vi "Pack for gRPC.vi"(8 "error in":errorcluster, 9 "configuration / results":enum16{"Configuration", "Results"}(ring), 10 "data value":variant, 11 "measurement plugin in":refnum<class "FPT Intermodulation.lvclass">) -> (0 "error out":errorcluster, 2 "any":T1, 3 "measurement plugin out":refnum<class "FPT Intermodulation.lvclass">)   [LabVIEW 2023, in "FPT Intermodulation.lvclass"]
uses:
  FPT Intermodulation.lvclass
  <vilib>/gRPC/LabVIEW gRPC Library/Shared/Any.ctl
  C:/Program Files/National Instruments/LabVIEW 2023/vi.lib/Plug-In SDKs/Measurements/Measurement Plugin Service/Measurement Plugin Service.lvclass
  Measurement Configuration.ctl
  Measurement Results.ctl
  2eca732d-dbaa-43bf-a7dd-ede2da65bc1b.vi
  a6012965-5700-4384-8228-972e71b6560c.vi
  <vilib>/gRPC/LabVIEW gRPC Library/Server API/Translate Protobuf Error.vi
  <vilib>/AdvancedString/1D String Array to Delimited String.vi
  <vilib>/gRPC/LabVIEW gRPC Library/Server API/Server/Get Server DLL Path.vi
  <vilib>/Plug-In SDKs/Measurements/Measurement Plugin Service/Measurement Plugin Service.lvclass
  <vilib>/gRPC/LabVIEW gRPC Library/grpc-lvsupport-release.lvlib
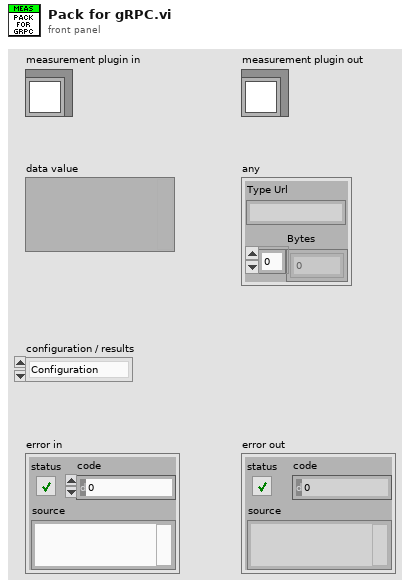
[diagram p1: front panel]
types:
  T1 = typedef "grpc-lvsupport-release.lvlib/Any.ctl" = cluster{"Type Url":string, "Bytes":u8[]}
  T2 = typedef "grpc-lvsupport-release.lvlib/grpcId.ctl" = u64
  T3 = typedef "FPT Intermodulation.lvclass/Measurement Configuration.ctl" = cluster{"Automation Test":bool, "Power sequencing file path":string, "RFSG name":string, "RFSG port":string, "RFSG attenuation mode":enum32{"<None>", "Constant Attenuation", "s2p File"}, "RFSG external attenuation (dB)":dbl, "RFSG s-parameters orientation":enum32{"Port1 Towards DUT", "Port2 Towards DUT"}, "RFSG s2p file path":string, "RFmx name":string, "RFmx port":string, "RFmx attenuation mode":enum32{"<None>", "Constant Attenuation", "s2p File"}, "RFmx external attenuation (dB)":dbl, "RFmx s-parameters orientation":enum32{"Port1 Towards DUT", "Port2 Towards DUT"}, "RFmx s2p file path":string, "RFmx Reference Level (dBm)":dbl, "RFSG Generation IQ Rate (S/s)":dbl, "Target Pout Per Tone (dBm)":dbl, "Start Pin Per Tone (dBm)":dbl, "Start Center Frequency (Hz)":dbl, "Start Tone Spacing (Hz)":dbl, "IM_Sweep Mode":enum32{"Power", "Frequency", "Tone Spacing"}, "Sweep Delay (ms)":u32, "Power Sweep End":dbl, "Power Sweep Step":dbl, "Frequency Sweep End":dbl, "Frequency Sweep Step":dbl, "Tone Spacing Sweep End":dbl, "Tone Spacing Sweep Step":dbl}
  T4 = typedef "FPT Intermodulation.lvclass/Measurement Results.ctl" = cluster{"Status":string, "Typical OIP3 (dBm)":dbl, "TS_Fundamental (dBm)":dbl[][], "TS_IMD (dBm)":dbl[][], "TS_TOI (dBm)":dbl[][], "TS_DUT Gain (dBm)":dbl[][], "Final Target Pout (dBm)":dbl}
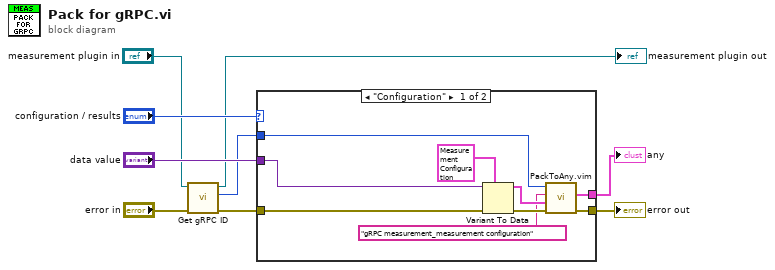
[diagram p0: block diagram]
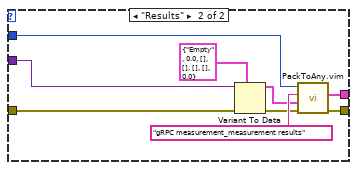
[diagram p2: hidden frame]
diagram:
  n1 = call <vilib>:"Get gRPC ID.vi"("error in"="error in", "measurement plugin service in"="measurement plugin in") -> ("error out"=w4:errorcluster, "gRPC ID"=w1:T2, "measurement plugin service out"=→"measurement plugin out":refnum<class "FPT Intermodulation.lvclass">)  [unwired: 7 in]
  n2 = case shown="\"Configuration\"" "configuration / results" {
    tunnel: w4 -> [w18 w27]
    tunnel: "data value" -> [w17 w26]
    tunnel: w1 -> [w14 w22]
    tunnel: [w16 w24] -> w8
    tunnel: [w15 w23] -> w7
    frame "Configuration" {
      n3 = Variant To Data(error in=w18, type=T3 {"Automation Test"=FALSE, "Power sequencing file path"="Lorem ipsum dolor sit", "RFSG name"="5842_0", "RFSG port"="", "RFSG attenuation mode"=enum."s2p File", "RFSG external attenuation (dB)"=1.2, "RFSG s-parameters orientation"=enum."Port1 Towards DUT", "RFSG s2p file path"="", "RFmx name"="5842_0", "RFmx port"="Lorem ipsum dolor sit", "RFmx attenuation mode"=enum."Constant Attenuation", "RFmx external attenuation (dB)"=1.0, "RFmx s-parameters orientation"=enum."Port2 Towards DUT", "RFmx s2p file path"="", "RFmx Reference Level (dBm)"=10.0, "RFSG Generation IQ Rate (S/s)"=1250000000.0, "Target Pout Per Tone (dBm)"=10.0, "Start Pin Per Tone (dBm)"=10.0, "Start Center Frequency (Hz)"=10.0, "Start Tone Spacing (Hz)"=10.0, "IM_Sweep Mode"=enum."Power", "Sweep Delay (ms)"=10, "Power Sweep End"=10.0, "Power Sweep Step"=10.0, "Frequency Sweep End"=-4.0, "Frequency Sweep Step"=1.0, "Tone Spacing Sweep End"=-4.0, "Tone Spacing Sweep Step"=1.0} ("measurement configuration"), Variant=w17) -> (data=w13:T3, error out=w12:errorcluster)
      n4 = call "PackToAny.vim"("error in"=w12, "Data To Pack"=w13, "Message Type"="gRPC measurement_measurement configuration", "gRPCid in"=w14) -> ("error out"=w16:errorcluster, "Any"=w15:T1)  [unwired: 5 in, 1 out]
    }
    frame "Results" {
      n5 = Variant To Data(error in=w27, type=T4 {"Status"="Empty", "Typical OIP3 (dBm)"=0.0, "TS_Fundamental (dBm)"=[], "TS_IMD (dBm)"=[], "TS_TOI (dBm)"=[], "TS_DUT Gain (dBm)"=[], "Final Target Pout (dBm)"=0.0} ("Measurement Results"), Variant=w26) -> (data=w20:T4, error out=w19:errorcluster)
      n6 = call "PackToAny.vim"("error in"=w19, "Data To Pack"=w20, "Message Type"="gRPC measurement_measurement results", "gRPCid in"=w22) -> ("error out"=w24:errorcluster, "Any"=w23:T1)  [unwired: 5 in, 1 out]
    }
  }
  "error out" <- w8
  "any" <- w7
